vi "ToString.vi"(8 "error in (no error)":errorcluster, 11 "IsRefnum in":refnum<class "IsRefnum.lvclass">) -> (0 "error out":errorcluster, 2 "String":string, 3 "IsRefnum out":refnum<class "IsRefnum.lvclass">)   [LabVIEW 2017, in "Transparent Assertions.lvlib" / "IsRefnum.lvclass"]
doc: "Returns a string representation of the object."
uses:
  IsRefnum.lvclass
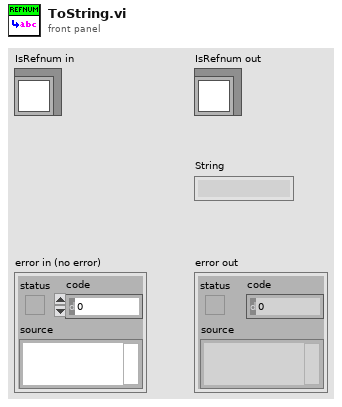
[diagram p1: front panel]
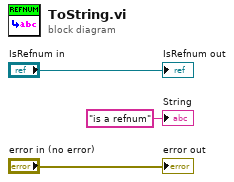
[diagram p0: block diagram]
diagram:
  "error out" <- "error in (no error)"
  "IsRefnum out" <- "IsRefnum in"
  "String" <- "is a refnum" ("String")
